vi "Main menu_3_enablepp.vi"() -> ()   [LabVIEW 2022 SP3]
uses:
  <vilib>/event_ctls.llb/lveventtype.ctl
  <vilib>/Utility/file.llb/Write Delimited Spreadsheet (DBL).vi
panel:
  in  "signal show":string(combo)
  out "Close":bool
  in  "Close app":bool
  out "Waveform Graph 2":waveform(sgl)(graph)
  in  "?":T1(tab)
  in  "New plot":bool
  in  "Multicolumn Listbox":i32(listbox)
  in  "Close All plots":bool
  in  "CSV":bool
  in  "Start":bool
  in  "Refresh time (ms)":i32
  in  "Mode":enum32{"Item 0", "Item 1"}(radio)
  in  "Size bytes":i32
  in  "Trace names":string(combo)
  out "Total\ncontrols":i32
  in  "# Control":string(combo)
  out "Current CS status":i32
  out "Enable?":bool
  in  "CS enable":bool
  in  "CS_IF_Cluster 2":T2 {"CS_Duty" min=0 max=1 scale=0.0..1.0}
  out "IP Free?":bool
  out "Server Ping":string
  out "Saved":bool
  in  "Save conf":bool
  in  "Ping IP":bool
  in  "Port":i32
  in  "hostname":string
  in  "timeout ms":i32
  in  "Send message":bool
  in  "Process 2":i32
  in  "msj":string
  # "hostname: 127.0.0.1\nport: 8085"
  # "hostname\n131.246.75.169"
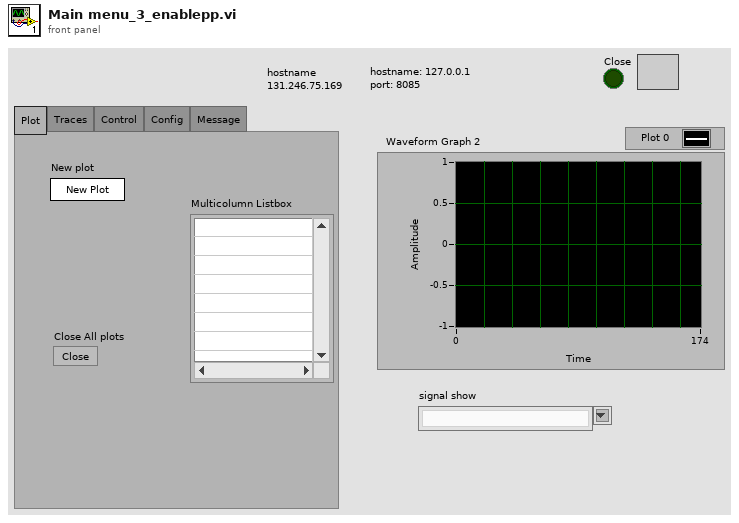
[diagram p1: front panel]
types:
  T1 = enum32{"Plot", "Traces", "Control", "Config", "Message"}
  T2 = cluster{"SET_DAMMS":i32, "CTLR":i32, "CS_Duty":sgl, "CS_IF_SET":i32}
  T3 = cluster{"Port":i32, "hostname":string, "status":bool, "timeout ms":i32, "TRACES_NAMES":string[], "Refresh time ms":i32, "Mode":enum32{"Item 0", "Item 1"}, "Start":bool, "DATA":sgl[][], "SIGNALS_NAMES":string[], "NB_SIGNALS":i32, "NB_TRACES":i32, "ID_TRACE":i32, "Mark":bool, "Counter":i32, "NAMES CSs":string[], "NB_CSs":i32}
  T4 = enum8{"Enabled", "Disabled", "Disabled and Grayed Out"}
  T5 = cluster{"TRACE_SIZE":i32, "CS_ID":i32, "TRACE ID":i32, "CMD":i32, "DATA(M)":i32}
  T6 = cluster{"timeout ms":i32, "remote port":u16, "Address":string}
  T7 = typedef "lveventtype.ctl" = enum32{"Null", "Timeout", "Annotation Menu Selection", "Annotation Menu Selection?", "App Instance Close", "App Instance Close?", "Autoscale Range Change", "Bookmark Info Change", "Cell Edit", "Cell Edit?", "Cursor Grab", "Cursor Grab?", "Cursor Menu Selection", "Cursor Menu Selection?", "Cursor Move", "Cursor Release", "Data Change", "Direction Change", "Display State Change", "Drag Ended", "Drag Enter", "Drag Leave", "Drag Over", "Drag Source Update", "Drag Starting", "Drag Starting?", "Drop", "Exec State Change", "Key Down", "Key Down?", "Key Repeat", "Key Repeat?", "Key Up", "Listbox Double Click", "Menu Activation?", "Menu Selection (App)", "Menu Selection? (App)", "Menu Selection (User)", "Mouse Down", "Mouse Down?", "Mouse Enter", "Mouse Leave", "Mouse Move", "Mouse Up", "Mouse Wheel", "NI Security User Change (App)", "Pane Size", "Panel Close", "Panel Close?", "Panel Resize", "Plot Attribute Change", "Scale Range Change", "Shortcut Menu Activation?", "Shortcut Menu Selection (App)", "Shortcut Menu Selection? (App)", "Shortcut Menu Selection (User)", "Tree Double Click", "Tree Drag", "Tree Drag?", "Tree Drop", "Tree Drop?", "Tree Item Close", "Tree Item Close?", "Tree Item Open", "Tree Item Open?", "User Event", "Value Change"}
  T8 = enum16{"open", "replace", "create", "open or create", "replace or create", "replace or create with confirmation"}
  T9 = cluster{"SIZE":i32, " TRACE DATA":sgl[], "TRACE_SIZE":i32, "NB_TRACES":i32, "NB_TRACED_SIGNALS":i32, "NAMES TRACED SIGNALS":string[], "NAMES TRACES":string[], "CS STATUS":i32, "NB_CSs":i32, "NAMES CSs":string[], "DATA (M)":sgl[], "CMD":i32}
  T10 = cluster{"SIZE":i32, "DATA":sgl[], "TRACE_SIZE":i32, "NB_TRACES":i32, "NB_SIGNALS":i32, "string":string[]}
  T11 = enum32{"invalid app kind", "Development System", "Run Time System", "Student Edition", "Embedded LabVIEW", "Evaluation", "Custom"}
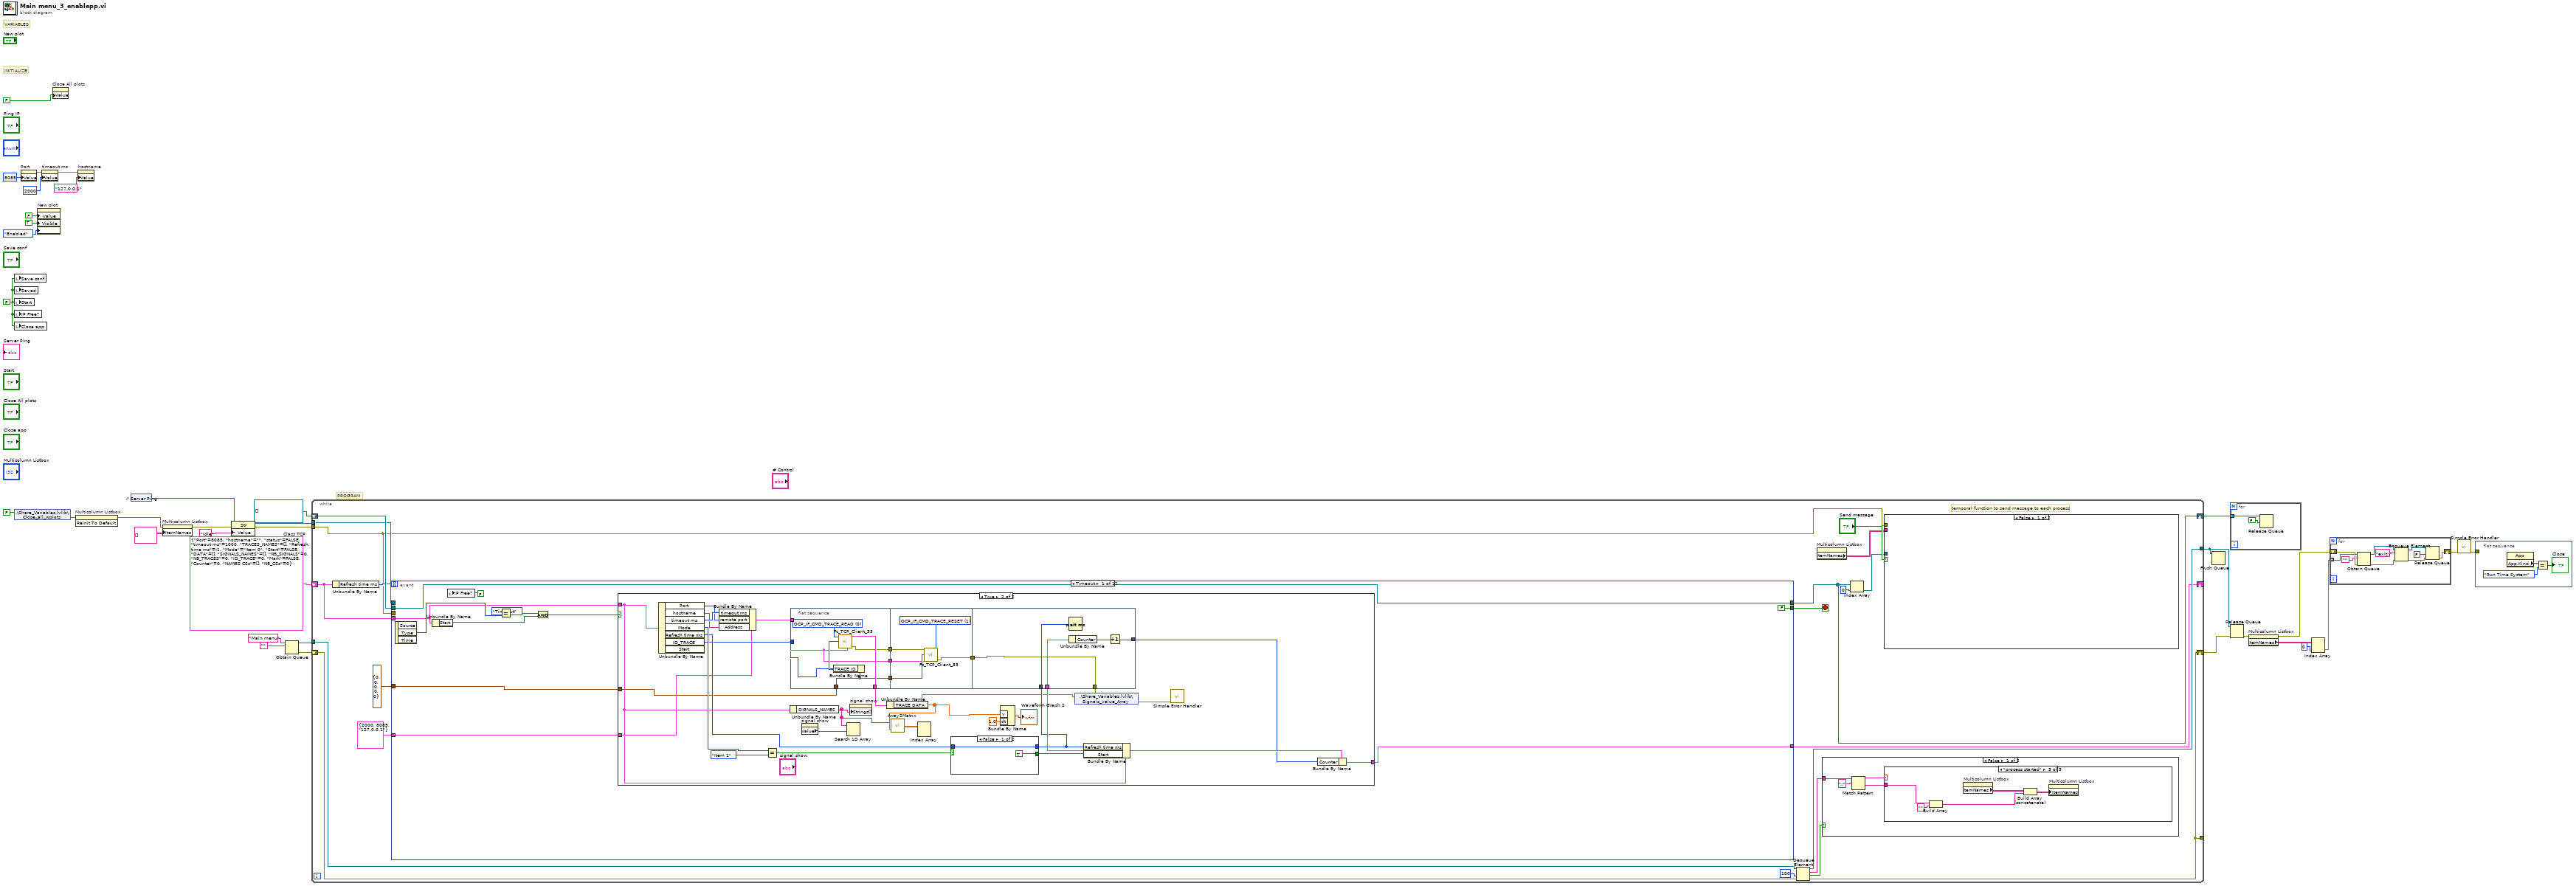
[diagram p0: block diagram]
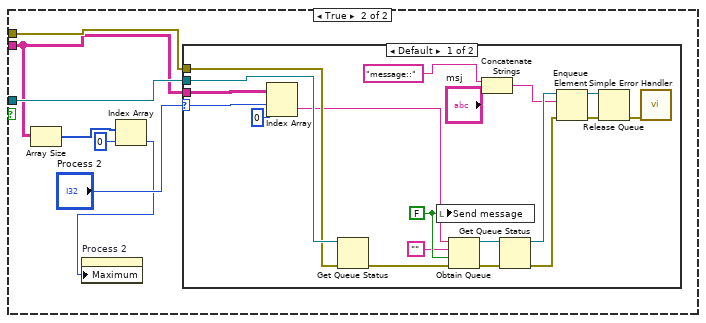
[diagram p2: hidden frame]
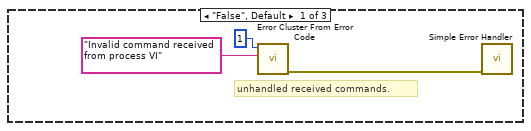
[diagram p4: hidden frame]
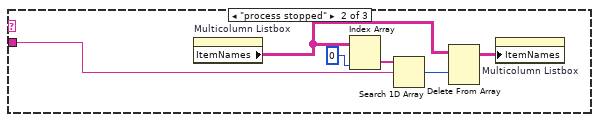
[diagram p5: hidden frame]
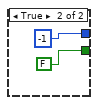
[diagram p8: hidden frame]
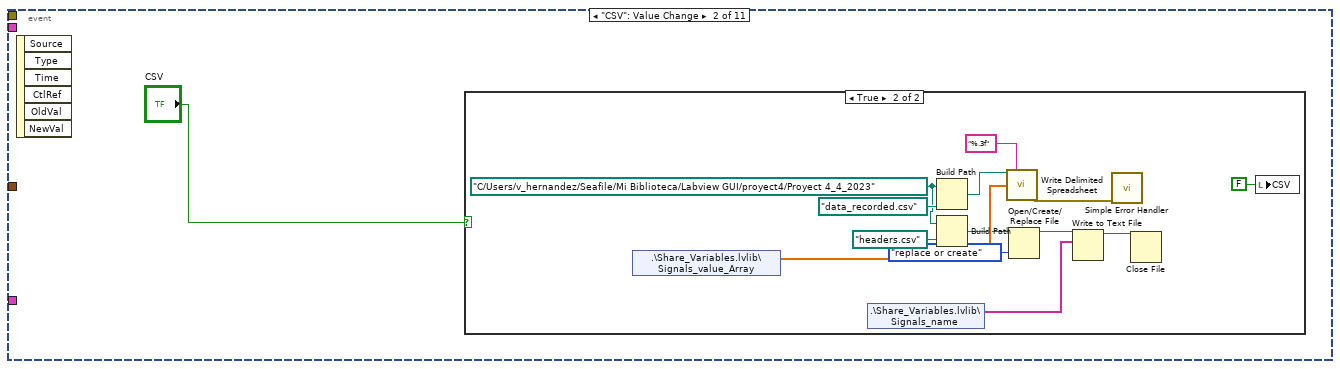
[diagram p9: hidden frame]
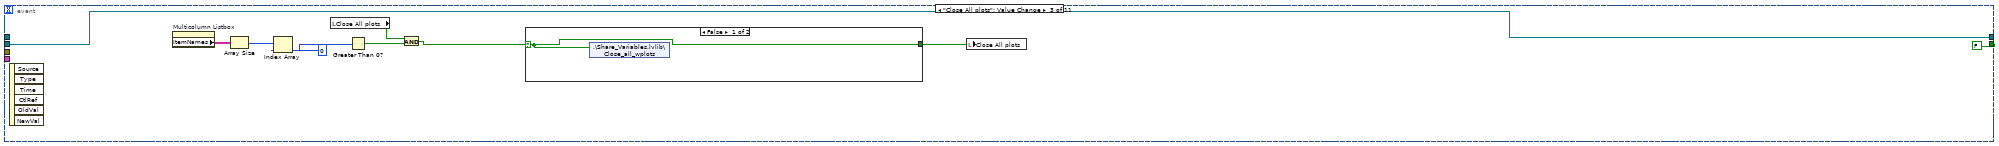
[diagram p11: hidden frame]
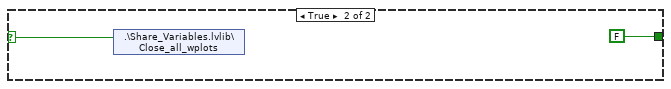
[diagram p12: hidden frame]
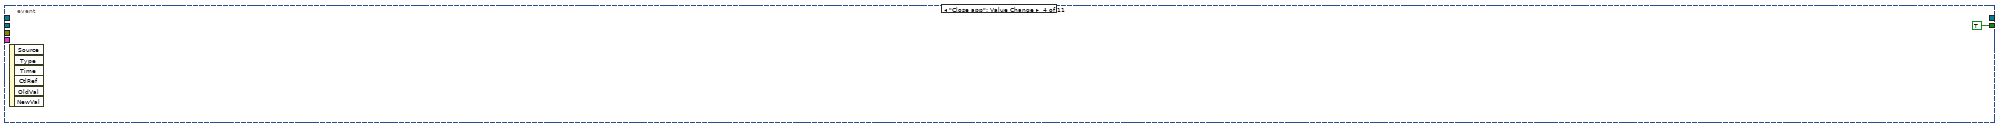
[diagram p13: hidden frame]
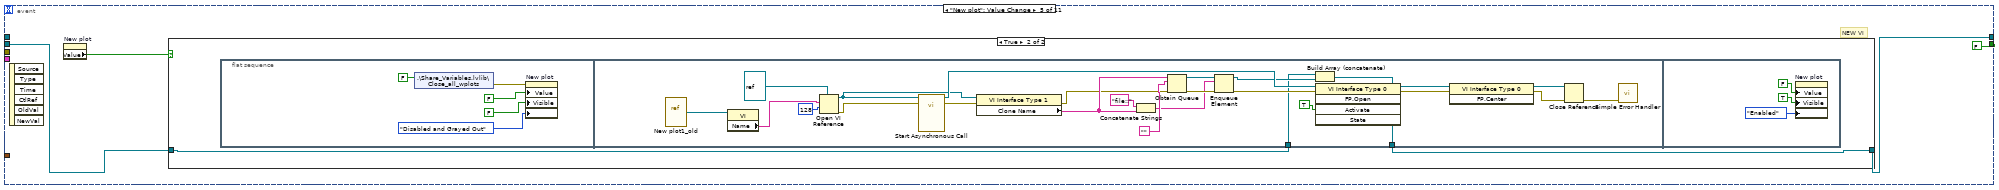
[diagram p14: hidden frame]
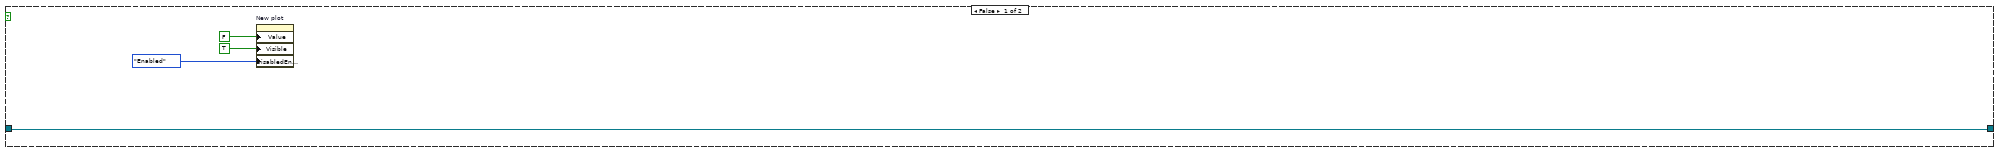
[diagram p15: hidden frame]
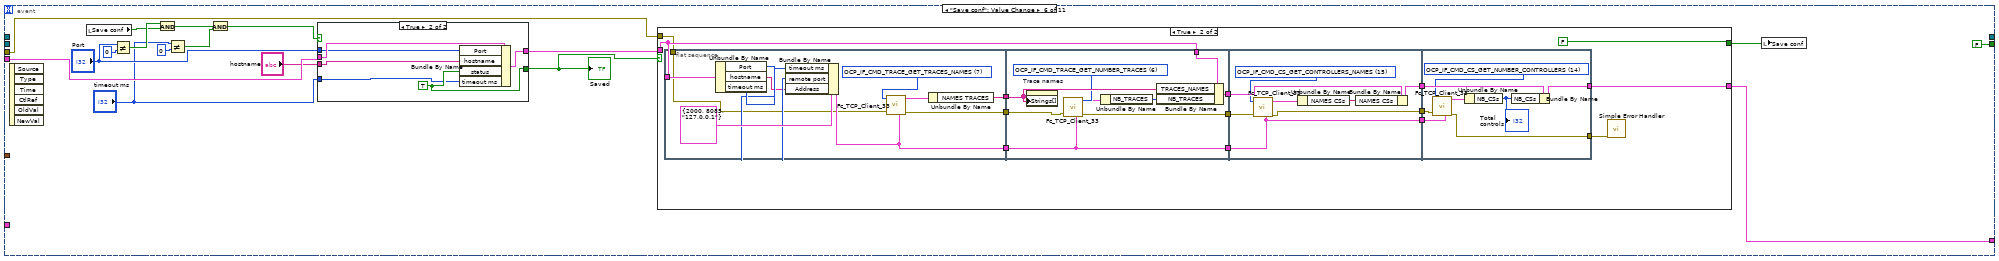
[diagram p16: hidden frame]
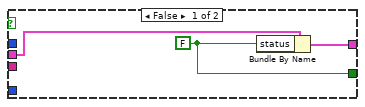
[diagram p18: hidden frame]
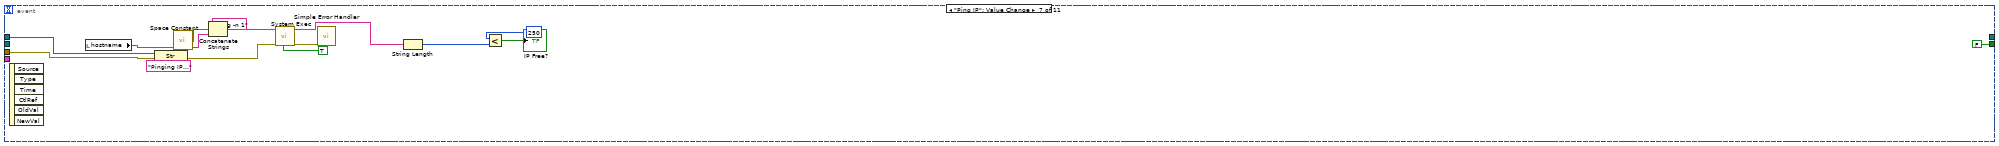
[diagram p19: hidden frame]
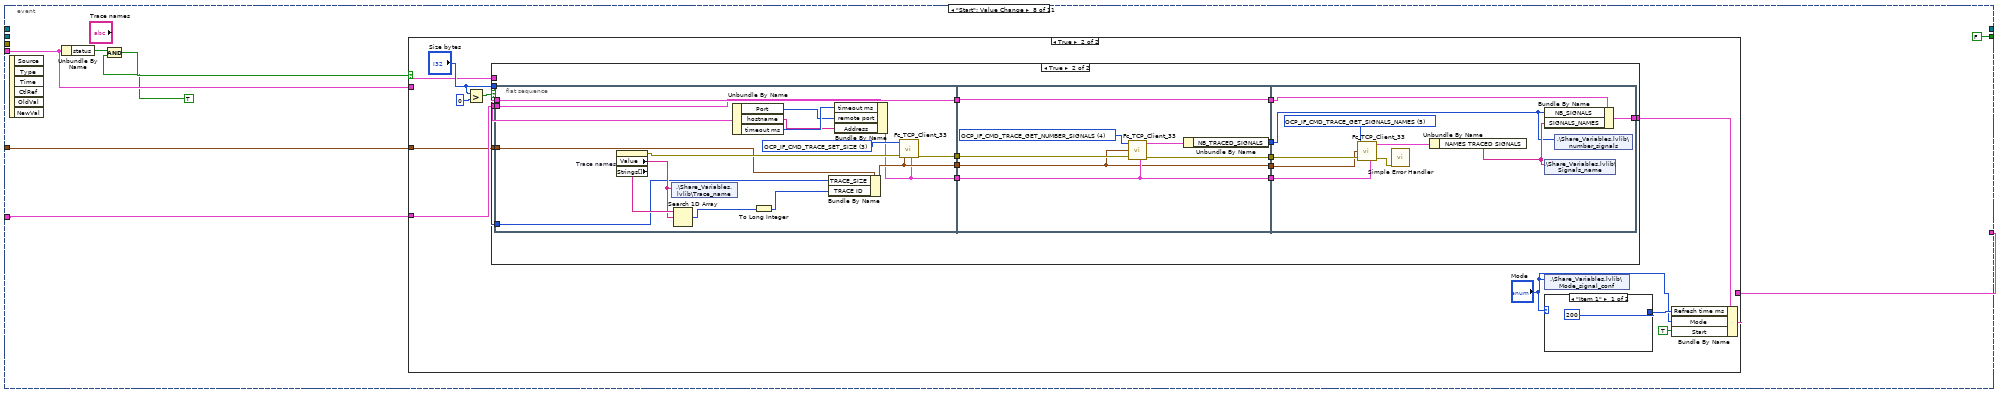
[diagram p20: hidden frame]
diagram:
  w13 = T3 {"Port"=8085, "hostname"="", "status"=FALSE, "timeout ms"=1000, "TRACES_NAMES"=[], "Refresh time ms"=-1, "Mode"=enum."Item 0", "Start"=FALSE, "DATA"=[], "SIGNALS_NAMES"=[], "NB_SIGNALS"=0, "NB_TRACES"=0, "ID_TRACE"=0, "Mark"=FALSE, "Counter"=0, "NAMES CSs"=[], "NB_CSs"=0}  # Class TCP
  w1 = FALSE ("Save conf")
  # "PROGRAM"
  # "INITIALIZE"
  # "VARIABLES"
  n1 = local write "Save conf"(w1) -> ()
  n2 = local write "Saved"(w1) -> ()
  n3 = local write "Start"(w1) -> ()
  n4 = local write "IP Free?"(w1) -> ()
  n5 = local write "Close app"(w1) -> ()
  n6 = shared-variable ".\\Share_Variables.lvlib\\Close_all_wplots"(FALSE ("Close_all_wplots")) -> (error out=w7:errorcluster)  [unwired: 1 in]
  n7 = property on="Port" class="DigNum (strict)"("Value"=8085) -> (error out=w8:errorcluster)  [unwired: 2 in, 1 out]
  n8 = property on="New plot" class="Bool (strict)"("Value"=FALSE ("New plot"), "Visible"=TRUE, "DisabledEnum"=T4."Enabled" ("Disabled")) -> ()  [unwired: 2 in, 2 out]
  n9 = property on="timeout ms" class="DigNum (strict)"(error in=w8, "Value"=2000 ("timeout ms")) -> (error out=w4:errorcluster)  [unwired: 1 in, 1 out]
  n10 = property on="Close All plots" class="Bool (strict)"("Value"=FALSE ("Cancel Button")) -> ()  [unwired: 2 in, 2 out]
  n11 = invoke on="Multicolumn Listbox" class="MCListbox (strict)" method="Reinit To Default"(error in=w7) -> (error out=w16:errorcluster)  [unwired: 2 in, 2 out]
  n12 = property on="hostname" class="Str"(error in=w4, "Value"="127.0.0.1" ("hostname")) -> ()  [unwired: 1 in, 2 out]
  n13 = control-ref of="Server Ping"() -> (w10:refnum<vi>)
  n14 = property on="Multicolumn Listbox" class="MCListbox (strict)"(error in=w16, "ItemNames"=string[][] [] ("Item Names")) -> (error out=w2:errorcluster)  [unwired: 1 in, 1 out]
  n15 = property class="Str"(reference=w10, error in=w2, "Value"="Idle" ("Ping status")) -> (reference out=w12:refnum<vi>, error out=w11:errorcluster)
  n16 = Obtain Queue(name (unnamed)="Main menu", element data type="") -> (queue out=w28:refnum<queue>, error out=w26:errorcluster)  [unwired: 3 in, 1 out]
  n17 = while {
    shift-right: [w39] -> w32
    shift-left: refnum<queue>[] [] -> [w55]
    tunnel: w28 -> [w54]
    tunnel: [w51] -> w18
    shift-right: [w44] -> w27
    shift-left: w26 -> [w50]
    shift-right: [w48] -> _
    shift-left: w13 -> [w46]
    tunnel: w12 -> [w47]
    tunnel: w11 -> [w41]
    tunnel: [w44] -> _
    stop <- w56 stop-if-true
    # "temporal function to send message to each process"
    n18 = Unbundle By Name(w46) -> ("Refresh time ms"=w45:i32)
    n19 = event shown="[0] Timeout" {
      selector: _ -> [_ _ _ _ _ _ _ _ _ _ _]
      dyn-events: _ -> [_ _ _ _ _ _ _ _ _ _ _]
      timeout: w45 -> [_ _ _ _ _ _ _ _ _ _ _]
      tunnel: [FALSE ("f") _ FALSE ("f") TRUE ("f") FALSE ("f") FALSE ("f") FALSE ("f") FALSE ("f") FALSE ("f") _ _] -> w56
      tunnel: [w112 _ w188 _ w195 _ _ _ _ _ _] -> w39
      tunnel: w55 -> [w112 _ w188 _ w194 _ _ _ _ _ _]
      tunnel: [w104 _ _ _ _ w242 _ w333 _ _ _] -> w48
      tunnel: w46 -> [w105 _ _ _ _ w250 _ w334 w414 w422 w446]
      tunnel: w47 -> [_ _ _ _ _ _ w328 _ _ _ _]
      tunnel: w41 -> [_ _ _ _ _ w245 w315 _ _ _ _]
      tunnel: T6 {"timeout ms"=2000, "remote port"=8085, "Address"="127.0.0.1"} ("Comunication Cluster") -> [w101 _ _ _ _ _ _ w330 _ w421 w445]
      tunnel: T5 {"TRACE_SIZE"=0, "CS_ID"=0, "TRACE ID"=0, "CMD"=0, "DATA(M)"=0} ("Input Cluster") -> [w102 _ _ _ _ _ _ w329 _ w420 w444]
      event Timeout {
        n20 = event-data() -> ("Type"=w109:T7)  [unwired: 1 in, 2 out]
        n21 = Unbundle By Name(w105) -> ("Start"=w107:bool)
        n22 = local write "IP Free?"(FALSE ("IP Free?")) -> ()
        n23 = Equal?(x=lveventtype."Timeout" ("Type"), y=w109) -> (x = y?=w108:bool)
        n24 = And(x=w108, y=w107) -> (x .and. y?=w106:bool)
        n25 = case shown="True" w106 {
          tunnel: w105 -> [w113 w118]
          tunnel: [w113 w133] -> w104
          tunnel: w102 -> [_ w120]
          tunnel: w101 -> [_ w119]
          frame False {
          }
          frame True {
            n26 = Unbundle By Name(w118) -> ("Port"=w125:i32, "hostname"=w124:string, "timeout ms"=w126:i32, "Mode"=w143:enum32{"Item 0", "Item 1"}, "Refresh time ms"=w140:i32, "ID_TRACE"=w137:i32)  [unwired: 1 out]
            n27 = Bundle By Name(cluster=w119, "timeout ms"=w126, "remote port"=w125, "Address"=w124) -> (w123:T6)
            n28 = Equal?(x=w143, y=enum32{"Item 0", "Item 1"}."Item 1" ("Mode")) -> (x = y?=w141:bool)
            n29 = Unbundle By Name(w118) -> ("SIGNALS_NAMES"=w116:string[])
            n30 = flat-sequence {
              tunnel: w137 -> [w146]
              tunnel: [w150] -> w136
              tunnel: [w149] -> w135
              tunnel: w120 -> [w145]
              tunnel: [w145] -> w128
              tunnel: [w144] -> w127
              tunnel: w123 -> [w144]
              tunnel: w135 -> [w155]
              tunnel: w128 -> [w154]
              tunnel: w127 -> [w153]
              tunnel: [w151] -> w122
              tunnel: w134 -> [w160]
              tunnel: [w158] -> w132
              tunnel: w130 -> [w157]
              tunnel: w122 -> [w156]
              tunnel: [w156] -> w121
              frame #0 {
                w148 = 0 items=["OCP_IF_CMD_TRACE_READ", "OCP_IF_CMD_TRACE_RESET", "OCP_IF_CMD_TRACE_GET_SIZE", "OCP_IF_CMD_TRACE_SET_SIZE", "OCP_IF_CMD_TRACE_GET_NUMBER_SIGNALS", "OCP_IF_CMD_TRACE_GET_SIGNALS_NAMES", "OCP_IF_CMD_TRACE_GET_NUMBER_TRACES", "OCP_IF_CMD_TRACE_GET_TRACES_NAMES", "OCP_IF_CMD_TRACE_GET_ADDRESS", "OCP_IF_CMD_CS_STATUS", "OCP_IF_CMD_CS_ENABLE", "OCP_IF_CMD_CS_DISABLE", "OCP_IF_CMD_CS_CONTROLLER_IF", "OCP_IF_CMD_CS_HARDWARE_IF", "OCP_IF_CMD_CS_GET_NUMBER_CONTROLLERS", "OCP_IF_CMD_CS_GET_CONTROLLERS_NAMES", "OCP_IF_CMD_PLATFORM_ID", "OCP_IF_CMD_PLATFORM_IF", "OCP_IF_CMD_OPIL_UPDATE_MEASUREMENTS", "OCP_IF_CMD_OPIL_UPDATE_SIM_DATA", "OCP_IF_CMD_OPIL_RUN_CONTROL", "OCP_IF_CMD_OPIL_INITIALIZE_CONTROL", "OCP_IF_CMD_OPIL_GET_CONTROL", "OCP_IF_CMD_OPIL_GET_CONTROLLER_DATA", "OCP_IF_CMD_END"] ("CMD")
                n31 = Bundle By Name(cluster=w145, "TRACE ID"=w146) -> (w147:T5)
                n32 = call "Fc_TCP_Client_33.vi"("CMD"=w148, "Input Cluster"=w147, "Comunication Cluster"=w144) -> ("Output cluster"=w150:T9, "error out"=w149:errorcluster)  [unwired: 5 in, 1 out]
              }
              frame #1 {
                w152 = 1 items=["OCP_IF_CMD_TRACE_READ", "OCP_IF_CMD_TRACE_RESET", "OCP_IF_CMD_TRACE_GET_SIZE", "OCP_IF_CMD_TRACE_SET_SIZE", "OCP_IF_CMD_TRACE_GET_NUMBER_SIGNALS", "OCP_IF_CMD_TRACE_GET_SIGNALS_NAMES", "OCP_IF_CMD_TRACE_GET_NUMBER_TRACES", "OCP_IF_CMD_TRACE_GET_TRACES_NAMES", "OCP_IF_CMD_TRACE_GET_ADDRESS", "OCP_IF_CMD_CS_STATUS", "OCP_IF_CMD_CS_ENABLE", "OCP_IF_CMD_CS_DISABLE", "OCP_IF_CMD_CS_CONTROLLER_IF", "OCP_IF_CMD_CS_HARDWARE_IF", "OCP_IF_CMD_CS_GET_NUMBER_CONTROLLERS", "OCP_IF_CMD_CS_GET_CONTROLLERS_NAMES", "OCP_IF_CMD_PLATFORM_ID", "OCP_IF_CMD_PLATFORM_IF", "OCP_IF_CMD_OPIL_UPDATE_MEASUREMENTS", "OCP_IF_CMD_OPIL_UPDATE_SIM_DATA", "OCP_IF_CMD_OPIL_RUN_CONTROL", "OCP_IF_CMD_OPIL_INITIALIZE_CONTROL", "OCP_IF_CMD_OPIL_GET_CONTROL", "OCP_IF_CMD_OPIL_GET_CONTROLLER_DATA", "OCP_IF_CMD_END"] ("CMD")
                n33 = call "Fc_TCP_Client_33.vi"("CMD"=w152, "Input Cluster"=w154, "error in (no error)"=w155, "Comunication Cluster"=w153) -> ("error out"=w151:errorcluster)  [unwired: 4 in, 2 out]
              }
              frame #2 {
                n34 = Wait (ms)(milliseconds to wait=w157) -> ()  [unwired: 1 out]
                n35 = Unbundle By Name(w160) -> ("Counter"=w159:i32)
                n36 = Increment(x=w159) -> (x+1=w158:i32)
              }
            }
            n37 = property on="signal show" class="CmbBox"() -> ("Value"=w115:string)  [unwired: 2 in, 2 out]
            n38 = Search 1D Array(1D array=w116, element=w115) -> ()  [unwired: 1 in, 1 out]
            n39 = property on="signal show" class="CmbBox"("Strings[]"=w116) -> ()  [unwired: 2 in, 2 out]
            n40 = Unbundle By Name(w136) -> ("TRACE DATA"=w117:sgl[])
            n41 = call "Array2Matrix.vi"("Array"=w117, "Header"=w116) -> ("Array2D"=w114:sgl[][])
            n42 = Index Array(array=w114) -> ()  [unwired: 2 in, 1 out]
            n43 = case shown="False" w141 {
              tunnel: [TRUE FALSE] -> w139
              tunnel: [w161 i8 -1 ("t")] -> w130
              tunnel: w140 -> [w161 _]
              frame False {
              }
              frame True {
              }
            }
            n44 = Bundle By Name("Y"=w117, "dt"=1.0) -> (→"Waveform Graph 2":waveform(sgl))  [unwired: 1 in]
            n45 = shared-variable ".\\Share_Variables.lvlib\\Signals_value_Array"(w117, error in=w121) -> (error out=w138:errorcluster)
            n46 = Bundle By Name(cluster=w118, "Refresh time ms"=w130, "Start"=w139) -> (w134:T3)
            n47 = call <vilib>:"Simple Error Handler.vi"("error in (no error)"=w138) -> ()  [unwired: 4 in, 5 out]
            n48 = Bundle By Name(cluster=w134, "Counter"=w132) -> (w133:T3)
          }
        }
      }
      event "CSV": Value Change {
        n49 = event-data() -> ()  [unwired: 1 in, 6 out]
        n50 = case shown="True" "CSV" {
          frame False {
          }
          frame True {
            w173 = path "C:/Users/v_hernandez/Seafile/Mi Biblioteca/Labview GUI/proyect4/Proyect 4_4_2023" ("base path")
            n51 = shared-variable ".\\Share_Variables.lvlib\\Signals_value_Array"() -> (w175:dbl[])  [unwired: 1 in, 1 out]
            n52 = shared-variable ".\\Share_Variables.lvlib\\Signals_name"() -> (w168:string[])  [unwired: 1 in, 1 out]
            n53 = Build Path(base path=w173, name or relative path=path "data_recorded.csv") -> (appended path=w174:path)
            n54 = Build Path(base path=w173, name or relative path=path "headers.csv") -> (appended path=w171:path)
            n55 = call-poly <vilib>:"Write Delimited Spreadsheet.vi"("file path (dialog if empty)"=w174, "format (%.3f)"="%.3f", "1D data"=w175) -> ("error out"=w176:errorcluster)  [unwired: 11 in, 1 out]
            n56 = Open/Create/Replace File(file path (use dialog)=w171, operation (0:open)=T8."replace or create") -> (refnum out=w169:refnum<file>)  [unwired: 4 in, 2 out]
            n57 = Write to Text File(file (use dialog)=w169, text=w168) -> (refnum out=w167:refnum<file>)  [unwired: 2 in, 2 out]
            n58 = call <vilib>:"Simple Error Handler.vi"("error in (no error)"=w176) -> ()  [unwired: 4 in, 5 out]
            n59 = Close File(refnum=w167) -> ()  [unwired: 1 in, 2 out]
            n60 = local write "CSV"(FALSE ("CSV")) -> ()
          }
        }
      }
      event "Close All plots": Value Change {
        n61 = event-data() -> ()  [unwired: 1 in, 6 out]
        n62 = property on="Multicolumn Listbox" class="MCListbox (strict)"() -> ("ItemNames"=w182:string[][])  [unwired: 2 in, 2 out]
        n63 = Array Size(array=w182) -> (size(s)=w186:i32[])
        n64 = Index Array(array=w186, index=0) -> (element=w184:i32)
        n65 = local read "Close All plots"() -> (w181:bool)
        n66 = Greater Than 0?(x=w184) -> (x > 0?=w179:bool)
        n67 = And(x=w181, y=w179) -> (x .and. y?=w180:bool)
        n68 = case shown="False" w180 {
          selector: w180 -> [w189 w190]
          tunnel: [w189 FALSE] -> w183
          frame False {
            n69 = shared-variable ".\\Share_Variables.lvlib\\Close_all_wplots"(w189) -> ()  [unwired: 1 in, 1 out]
          }
          frame True {
            n70 = shared-variable ".\\Share_Variables.lvlib\\Close_all_wplots"(w190) -> ()  [unwired: 1 in, 1 out]
          }
        }
        n71 = local write "Close All plots"(w183) -> ()
      }
      event "Close app": Value Change {
        n72 = event-data() -> ()  [unwired: 1 in, 6 out]
      }
      event "New plot": Value Change {
        # "NEW VI"
        n73 = event-data() -> ()  [unwired: 1 in, 6 out]
        n74 = property on="New plot" class="Bool (strict)"() -> ("Value"=w196:bool)  [unwired: 2 in, 2 out]
        n75 = case shown="True" w196 {
          tunnel: [w197 w202] -> w195
          tunnel: w194 -> [w197 w201]
          frame False {
            n76 = property on="New plot" class="Bool (strict)"("Value"=FALSE ("New plot"), "Visible"=TRUE, "DisabledEnum"=T4."Enabled" ("Disabled")) -> ()  [unwired: 2 in, 2 out]
          }
          frame True {
            n77 = flat-sequence {
              tunnel: [w213] -> w202
              tunnel: w201 -> [w212]
              frame #0 {
                n78 = shared-variable ".\\Share_Variables.lvlib\\Close_all_wplots"(FALSE ("Close_all_wplots")) -> (error out=w203:errorcluster)  [unwired: 1 in]
                n79 = property on="New plot" class="Bool (strict)"(error in=w203, "Value"=FALSE ("New plot"), "Visible"=FALSE, "DisabledEnum"=T4."Disabled and Grayed Out" ("Disabled")) -> ()  [unwired: 1 in, 2 out]
              }
              frame #1 {
                n80 = vi-ref "New plot1_old.vi"() -> (w226:refnum<vi>)
                n81 = property class="VI"(reference=w226) -> ("Name"=w232:string)  [unwired: 1 in, 2 out]
                n82 = Open VI Reference(type specifier VI Refnum (for type only)=refnum<vi> refnum, vi path=w232, options=128) -> (vi reference=w223:refnum<vi>, error out=w228:errorcluster)  [unwired: 3 in]
                n83 = call-by-ref "Start Asynchronous Call"(reference=w223, error in=w228) -> (reference out=w227:refnum<vi>, error out=w217:errorcluster)  [unwired: 1 in, 1 out]
                n84 = property class="VI Interface Type 1"(reference=w223, error in=w217) -> (error out=w218:errorcluster, "Clone Name"=w220:string)  [unwired: 1 out]
                n85 = Concatenate Strings("file::" ("string"), w220) -> (w211:string)
                n86 = Obtain Queue(name (unnamed)=w220, element data type="", error in (no error)=w218) -> (queue out=w219:refnum<queue>, error out=w216:errorcluster)  [unwired: 2 in, 1 out]
                n87 = Enqueue Element(queue=w219, element=w211, error in (no error)=w216) -> (queue out=w214:refnum<queue>, error out=w215:errorcluster)  [unwired: 1 in, 1 out]
                n88 = Build Array (concatenate)(w212, w214) -> (w213:refnum<queue>[])
                n89 = invoke class="VI Interface Type 0" method="FP.Open"(reference=w227, error in=w215, "Activate"=TRUE ("Activate?")) -> (reference out=w225:refnum<vi>, error out=w210:errorcluster)  [unwired: 2 in, 3 out]
                n90 = invoke class="VI Interface Type 0" method="FP.Center"(reference=w225, error in=w210) -> (reference out=w224:refnum<vi>, error out=w209:errorcluster)  [unwired: 1 in, 1 out]
                n91 = Close Reference(reference=w224, error in (no error)=w209) -> (error out=w208:errorcluster)
                n92 = call <vilib>:"Simple Error Handler.vi"("error in (no error)"=w208) -> ()  [unwired: 4 in, 5 out]
              }
              frame #2 {
                n93 = property on="New plot" class="Bool (strict)"("Value"=FALSE ("Value (Signaling)"), "Visible"=TRUE, "DisabledEnum"=T4."Enabled" ("Disabled")) -> ()  [unwired: 2 in, 2 out]
              }
            }
          }
        }
      }
      event "Save conf": Value Change {
        n94 = event-data() -> ()  [unwired: 1 in, 6 out]
        n95 = local read "Save conf"() -> (w247:bool)
        n96 = Not Equal?(x="Port", y=0) -> (x != y?=w251:bool)
        n97 = And(x=w251, y=w247) -> (x .and. y?=w237:bool)
        n98 = Not Equal?(x="timeout ms", y=0) -> (x != y?=w239:bool)
        n99 = And(x=w237, y=w239) -> (x .and. y?=w238:bool)
        n100 = case shown="True" w238 {
          tunnel: [w305 w310] -> w246
          tunnel: "Port" -> [_ w312]
          tunnel: "hostname" -> [_ w311]
          tunnel: [w307 w308] -> w243
          tunnel: w250 -> [w306 w313]
          tunnel: "timeout ms" -> [_ w309]
          frame False {
            w305 = FALSE
            n101 = Bundle By Name(cluster=w306, "status"=w305) -> (w307:T3)
          }
          frame True {
            w310 = TRUE
            n102 = Bundle By Name(cluster=w313, "Port"=w312, "hostname"=w311, "status"=w310, "timeout ms"=w309) -> (w308:T3)
          }
        }
        "Saved" <- w246
        n103 = case shown="True" w246 {
          selector: w246 -> [w253 _]
          tunnel: w245 -> [_ w256]
          tunnel: [w253 FALSE] -> w244
          tunnel: w243 -> [w254 w267]
          tunnel: [w254 w266] -> w242
          frame False {
          }
          frame True {
            n104 = flat-sequence {
              tunnel: w267 -> [w279]
              tunnel: [w272] -> w265
              tunnel: [w271] -> w264
              tunnel: [w270] -> w263
              tunnel: w256 -> [w269]
              tunnel: w267 -> [w288]
              tunnel: w265 -> [w285]
              tunnel: w264 -> [w284]
              tunnel: w263 -> [w280]
              tunnel: [w287] -> w262
              tunnel: [w281] -> w260
              tunnel: [w280] -> w259
              tunnel: w262 -> [w296]
              tunnel: [w290] -> w261
              tunnel: w260 -> [w295]
              tunnel: w259 -> [w292]
              tunnel: [w293] -> w258
              tunnel: [w292] -> w257
              tunnel: [w300] -> w266
              tunnel: w261 -> [w304]
              tunnel: w258 -> [w303]
              tunnel: w257 -> [w302]
              tunnel: [w298] -> w255
              frame #0 {
                w278 = 7 items=["OCP_IF_CMD_TRACE_READ", "OCP_IF_CMD_TRACE_RESET", "OCP_IF_CMD_TRACE_GET_SIZE", "OCP_IF_CMD_TRACE_SET_SIZE", "OCP_IF_CMD_TRACE_GET_NUMBER_SIGNALS", "OCP_IF_CMD_TRACE_GET_SIGNALS_NAMES", "OCP_IF_CMD_TRACE_GET_NUMBER_TRACES", "OCP_IF_CMD_TRACE_GET_TRACES_NAMES", "OCP_IF_CMD_TRACE_GET_ADDRESS", "OCP_IF_CMD_CS_STATUS", "OCP_IF_CMD_CS_ENABLE", "OCP_IF_CMD_CS_DISABLE", "OCP_IF_CMD_CS_CONTROLLER_IF", "OCP_IF_CMD_CS_HARDWARE_IF", "OCP_IF_CMD_CS_GET_NUMBER_CONTROLLERS", "OCP_IF_CMD_CS_GET_CONTROLLERS_NAMES", "OCP_IF_CMD_PLATFORM_ID", "OCP_IF_CMD_PLATFORM_IF", "OCP_IF_CMD_OPIL_UPDATE_MEASUREMENTS", "OCP_IF_CMD_OPIL_UPDATE_SIM_DATA", "OCP_IF_CMD_OPIL_RUN_CONTROL", "OCP_IF_CMD_OPIL_INITIALIZE_CONTROL", "OCP_IF_CMD_OPIL_GET_CONTROL", "OCP_IF_CMD_OPIL_GET_CONTROLLER_DATA", "OCP_IF_CMD_END"] ("CMD")
                n105 = Unbundle By Name(w279) -> ("Port"=w274:i32, "hostname"=w273:string, "timeout ms"=w275:i32)
                n106 = Bundle By Name(cluster=T6 {"timeout ms"=2000, "remote port"=8085, "Address"="127.0.0.1"} ("Comunication Cluster"), "timeout ms"=w275, "remote port"=w274, "Address"=w273) -> (w270:T6)
                n107 = call "Fc_TCP_Client_33.vi"("CMD"=w278, "error in (no error)"=w269, "Comunication Cluster"=w270) -> ("Output cluster"=w277:T9, "error out"=w271:errorcluster)  [unwired: 5 in, 1 out]
                n108 = Unbundle By Name(w277) -> ("NAMES TRACES"=w272:string[])
              }
              frame #1 {
                w283 = 6 items=["OCP_IF_CMD_TRACE_READ", "OCP_IF_CMD_TRACE_RESET", "OCP_IF_CMD_TRACE_GET_SIZE", "OCP_IF_CMD_TRACE_SET_SIZE", "OCP_IF_CMD_TRACE_GET_NUMBER_SIGNALS", "OCP_IF_CMD_TRACE_GET_SIGNALS_NAMES", "OCP_IF_CMD_TRACE_GET_NUMBER_TRACES", "OCP_IF_CMD_TRACE_GET_TRACES_NAMES", "OCP_IF_CMD_TRACE_GET_ADDRESS", "OCP_IF_CMD_CS_STATUS", "OCP_IF_CMD_CS_ENABLE", "OCP_IF_CMD_CS_DISABLE", "OCP_IF_CMD_CS_CONTROLLER_IF", "OCP_IF_CMD_CS_HARDWARE_IF", "OCP_IF_CMD_CS_GET_NUMBER_CONTROLLERS", "OCP_IF_CMD_CS_GET_CONTROLLERS_NAMES", "OCP_IF_CMD_PLATFORM_ID", "OCP_IF_CMD_PLATFORM_IF", "OCP_IF_CMD_OPIL_UPDATE_MEASUREMENTS", "OCP_IF_CMD_OPIL_UPDATE_SIM_DATA", "OCP_IF_CMD_OPIL_RUN_CONTROL", "OCP_IF_CMD_OPIL_INITIALIZE_CONTROL", "OCP_IF_CMD_OPIL_GET_CONTROL", "OCP_IF_CMD_OPIL_GET_CONTROLLER_DATA", "OCP_IF_CMD_END"] ("CMD")
                n109 = property on="Trace names" class="CmbBox"("Strings[]"=w285) -> ()  [unwired: 2 in, 2 out]
                n110 = call "Fc_TCP_Client_33.vi"("CMD"=w283, "error in (no error)"=w284, "Comunication Cluster"=w280) -> ("Output cluster"=w282:T9, "error out"=w281:errorcluster)  [unwired: 5 in, 1 out]
                n111 = Unbundle By Name(w282) -> ("NB_TRACES"=w286:i32)
                n112 = Bundle By Name(cluster=w288, "TRACES_NAMES"=w285, "NB_TRACES"=w286) -> (w287:T3)
              }
              frame #2 {
                w294 = 15 items=["OCP_IF_CMD_TRACE_READ", "OCP_IF_CMD_TRACE_RESET", "OCP_IF_CMD_TRACE_GET_SIZE", "OCP_IF_CMD_TRACE_SET_SIZE", "OCP_IF_CMD_TRACE_GET_NUMBER_SIGNALS", "OCP_IF_CMD_TRACE_GET_SIGNALS_NAMES", "OCP_IF_CMD_TRACE_GET_NUMBER_TRACES", "OCP_IF_CMD_TRACE_GET_TRACES_NAMES", "OCP_IF_CMD_TRACE_GET_ADDRESS", "OCP_IF_CMD_CS_STATUS", "OCP_IF_CMD_CS_ENABLE", "OCP_IF_CMD_CS_DISABLE", "OCP_IF_CMD_CS_CONTROLLER_IF", "OCP_IF_CMD_CS_HARDWARE_IF", "OCP_IF_CMD_CS_GET_NUMBER_CONTROLLERS", "OCP_IF_CMD_CS_GET_CONTROLLERS_NAMES", "OCP_IF_CMD_PLATFORM_ID", "OCP_IF_CMD_PLATFORM_IF", "OCP_IF_CMD_OPIL_UPDATE_MEASUREMENTS", "OCP_IF_CMD_OPIL_UPDATE_SIM_DATA", "OCP_IF_CMD_OPIL_RUN_CONTROL", "OCP_IF_CMD_OPIL_INITIALIZE_CONTROL", "OCP_IF_CMD_OPIL_GET_CONTROL", "OCP_IF_CMD_OPIL_GET_CONTROLLER_DATA", "OCP_IF_CMD_END"] ("CMD")
                n113 = call "Fc_TCP_Client_33.vi"("CMD"=w294, "error in (no error)"=w295, "Comunication Cluster"=w292) -> ("Output cluster"=w291:T9, "error out"=w293:errorcluster)  [unwired: 5 in, 1 out]
                n114 = Unbundle By Name(w291) -> ("NAMES CSs"=w289:string[])
                n115 = Bundle By Name(cluster=w296, "NAMES CSs"=w289) -> (w290:T3)
              }
              frame #3 {
                w301 = 14 items=["OCP_IF_CMD_TRACE_READ", "OCP_IF_CMD_TRACE_RESET", "OCP_IF_CMD_TRACE_GET_SIZE", "OCP_IF_CMD_TRACE_SET_SIZE", "OCP_IF_CMD_TRACE_GET_NUMBER_SIGNALS", "OCP_IF_CMD_TRACE_GET_SIGNALS_NAMES", "OCP_IF_CMD_TRACE_GET_NUMBER_TRACES", "OCP_IF_CMD_TRACE_GET_TRACES_NAMES", "OCP_IF_CMD_TRACE_GET_ADDRESS", "OCP_IF_CMD_CS_STATUS", "OCP_IF_CMD_CS_ENABLE", "OCP_IF_CMD_CS_DISABLE", "OCP_IF_CMD_CS_CONTROLLER_IF", "OCP_IF_CMD_CS_HARDWARE_IF", "OCP_IF_CMD_CS_GET_NUMBER_CONTROLLERS", "OCP_IF_CMD_CS_GET_CONTROLLERS_NAMES", "OCP_IF_CMD_PLATFORM_ID", "OCP_IF_CMD_PLATFORM_IF", "OCP_IF_CMD_OPIL_UPDATE_MEASUREMENTS", "OCP_IF_CMD_OPIL_UPDATE_SIM_DATA", "OCP_IF_CMD_OPIL_RUN_CONTROL", "OCP_IF_CMD_OPIL_INITIALIZE_CONTROL", "OCP_IF_CMD_OPIL_GET_CONTROL", "OCP_IF_CMD_OPIL_GET_CONTROLLER_DATA", "OCP_IF_CMD_END"] ("CMD")
                n116 = call "Fc_TCP_Client_33.vi"("CMD"=w301, "error in (no error)"=w303, "Comunication Cluster"=w302) -> ("Output cluster"=w299:T9, "error out"=w298:errorcluster)  [unwired: 5 in, 1 out]
                n117 = Unbundle By Name(w299) -> ("NB_CSs"=w297:i32)
                "Total\ncontrols" <- w297
                n118 = Bundle By Name(cluster=w304, "NB_CSs"=w297) -> (w300:T3)
              }
            }
            n119 = call <vilib>:"Simple Error Handler.vi"("error in (no error)"=w255) -> ()  [unwired: 4 in, 5 out]
          }
        }
        n120 = local write "Save conf"(w244) -> ()
      }
      event "Ping IP": Value Change {
        n121 = event-data() -> ()  [unwired: 1 in, 6 out]
        n122 = local read "hostname"() -> (w323:string)
        n123 = property class="Str"(reference=w328, error in=w315, "Value"="Pinging IP...") -> (error out=w326:errorcluster)  [unwired: 1 out]
        n124 = call <vilib>:"Space Constant.vi"() -> ("String"=w324:string)
        n125 = Concatenate Strings("ping -n 1" ("Value"), w324, w323) -> (w322:string)
        n126 = call <vilib>:"System Exec.vi"("run minimized? (F)"=TRUE, "error in (no error)"=w326, "command line"=w322) -> ("error out"=w316:errorcluster, "standard output"=w320:string)  [unwired: 5 in, 2 out]
        n127 = call <vilib>:"Simple Error Handler.vi"("error in (no error)"=w316) -> ()  [unwired: 4 in, 5 out]
        n128 = String Length(string=w320) -> (length=w321:i32)
        n129 = Less?(x=250, y=w321) -> (x < y?=→"IP Free?":bool)
      }
      event "Start": Value Change {
        n130 = event-data() -> ()  [unwired: 1 in, 6 out]
        n131 = Unbundle By Name(w334) -> ("status"=w336:bool)
        n132 = And(x=w336, y=TRUE) -> (x .and. y?=w335:bool)
        n133 = case shown="True" w335 {
          tunnel: w334 -> [w337 w342]
          tunnel: [w337 w348] -> w333
          tunnel: w330 -> [_ w339]
          tunnel: w329 -> [_ w338]
          frame False {
          }
          frame True {
            n134 = Greater?(x="Size bytes", y=0) -> (0:w344:bool)
            n135 = case shown="True" w344 {
              tunnel: "Size bytes" -> [_ w363]
              tunnel: w342 -> [w349 w362]
              tunnel: [w349 w358] -> w341
              tunnel: w339 -> [_ w351]
              tunnel: w338 -> [_ w350]
              frame False {
              }
              frame True {
                n136 = flat-sequence {
                  tunnel: w363 -> [w369]
                  tunnel: w362 -> [w379]
                  tunnel: [w375] -> w361
                  tunnel: [w379] -> w360
                  tunnel: [w367] -> w357
                  tunnel: [w366] -> w356
                  tunnel: w351 -> [w365]
                  tunnel: w350 -> [w364]
                  tunnel: w361 -> [w386]
                  tunnel: w360 -> [w387]
                  tunnel: [w387] -> w359
                  tunnel: w357 -> [w380]
                  tunnel: w356 -> [w381]
                  tunnel: [w383] -> w355
                  tunnel: [w382] -> w354
                  tunnel: [w381] -> w353
                  tunnel: [w380] -> w352
                  tunnel: w359 -> [w397]
                  tunnel: [w396] -> w358
                  tunnel: w355 -> [w388]
                  tunnel: w354 -> [w392]
                  tunnel: w353 -> [w390]
                  tunnel: w352 -> [w389]
                  frame #0 {
                    w374 = 3 items=["OCP_IF_CMD_TRACE_READ", "OCP_IF_CMD_TRACE_RESET", "OCP_IF_CMD_TRACE_GET_SIZE", "OCP_IF_CMD_TRACE_SET_SIZE", "OCP_IF_CMD_TRACE_GET_NUMBER_SIGNALS", "OCP_IF_CMD_TRACE_GET_SIGNALS_NAMES", "OCP_IF_CMD_TRACE_GET_NUMBER_TRACES", "OCP_IF_CMD_TRACE_GET_TRACES_NAMES", "OCP_IF_CMD_TRACE_GET_ADDRESS", "OCP_IF_CMD_CS_STATUS", "OCP_IF_CMD_CS_ENABLE", "OCP_IF_CMD_CS_DISABLE", "OCP_IF_CMD_CS_CONTROLLER_IF", "OCP_IF_CMD_CS_HARDWARE_IF", "OCP_IF_CMD_CS_GET_NUMBER_CONTROLLERS", "OCP_IF_CMD_CS_GET_CONTROLLERS_NAMES", "OCP_IF_CMD_PLATFORM_ID", "OCP_IF_CMD_PLATFORM_IF", "OCP_IF_CMD_OPIL_UPDATE_MEASUREMENTS", "OCP_IF_CMD_OPIL_UPDATE_SIM_DATA", "OCP_IF_CMD_OPIL_RUN_CONTROL", "OCP_IF_CMD_OPIL_INITIALIZE_CONTROL", "OCP_IF_CMD_OPIL_GET_CONTROL", "OCP_IF_CMD_OPIL_GET_CONTROLLER_DATA", "OCP_IF_CMD_END"] ("CMD")
                    n137 = property on="Trace names" class="CmbBox"() -> (error out=w370:errorcluster, "Value"=w376:string, "Strings[]"=w378:string[])  [unwired: 2 in, 1 out]
                    n138 = shared-variable ".\\Share_Variables.lvlib\\Trace_name"(w376) -> ()  [unwired: 1 in, 1 out]
                    n139 = Search 1D Array(1D array=w378, element=w376) -> (index of element=w377:i32)  [unwired: 1 in]
                    n140 = Unbundle By Name(w379) -> ("Port"=w372:i32, "hostname"=w371:string, "timeout ms"=w373:i32)
                    n141 = To Long Integer(number=w377) -> (32bit integer=w368:i32)
                    n142 = Bundle By Name(cluster=w364, "TRACE_SIZE"=w369, "TRACE ID"=w368) -> (w367:T5)
                    n143 = Bundle By Name(cluster=w365, "timeout ms"=w373, "remote port"=w372, "Address"=w371) -> (w366:T6)
                    n144 = call "Fc_TCP_Client_33.vi"("CMD"=w374, "Input Cluster"=w367, "error in (no error)"=w370, "Comunication Cluster"=w366) -> ("error out"=w375:errorcluster)  [unwired: 4 in, 2 out]
                  }
                  frame #1 {
                    w385 = 4 items=["OCP_IF_CMD_TRACE_READ", "OCP_IF_CMD_TRACE_RESET", "OCP_IF_CMD_TRACE_GET_SIZE", "OCP_IF_CMD_TRACE_SET_SIZE", "OCP_IF_CMD_TRACE_GET_NUMBER_SIGNALS", "OCP_IF_CMD_TRACE_GET_SIGNALS_NAMES", "OCP_IF_CMD_TRACE_GET_NUMBER_TRACES", "OCP_IF_CMD_TRACE_GET_TRACES_NAMES", "OCP_IF_CMD_TRACE_GET_ADDRESS", "OCP_IF_CMD_CS_STATUS", "OCP_IF_CMD_CS_ENABLE", "OCP_IF_CMD_CS_DISABLE", "OCP_IF_CMD_CS_CONTROLLER_IF", "OCP_IF_CMD_CS_HARDWARE_IF", "OCP_IF_CMD_CS_GET_NUMBER_CONTROLLERS", "OCP_IF_CMD_CS_GET_CONTROLLERS_NAMES", "OCP_IF_CMD_PLATFORM_ID", "OCP_IF_CMD_PLATFORM_IF", "OCP_IF_CMD_OPIL_UPDATE_MEASUREMENTS", "OCP_IF_CMD_OPIL_UPDATE_SIM_DATA", "OCP_IF_CMD_OPIL_RUN_CONTROL", "OCP_IF_CMD_OPIL_INITIALIZE_CONTROL", "OCP_IF_CMD_OPIL_GET_CONTROL", "OCP_IF_CMD_OPIL_GET_CONTROLLER_DATA", "OCP_IF_CMD_END"] ("CMD")
                    n145 = call "Fc_TCP_Client_33.vi"("CMD"=w385, "Input Cluster"=w380, "error in (no error)"=w386, "Comunication Cluster"=w381) -> ("Output cluster"=w384:T9, "error out"=w382:errorcluster)  [unwired: 4 in, 1 out]
                    n146 = Unbundle By Name(w384) -> ("NB_TRACED_SIGNALS"=w383:i32)
                  }
                  frame #2 {
                    w391 = 5 items=["OCP_IF_CMD_TRACE_READ", "OCP_IF_CMD_TRACE_RESET", "OCP_IF_CMD_TRACE_GET_SIZE", "OCP_IF_CMD_TRACE_SET_SIZE", "OCP_IF_CMD_TRACE_GET_NUMBER_SIGNALS", "OCP_IF_CMD_TRACE_GET_SIGNALS_NAMES", "OCP_IF_CMD_TRACE_GET_NUMBER_TRACES", "OCP_IF_CMD_TRACE_GET_TRACES_NAMES", "OCP_IF_CMD_TRACE_GET_ADDRESS", "OCP_IF_CMD_CS_STATUS", "OCP_IF_CMD_CS_ENABLE", "OCP_IF_CMD_CS_DISABLE", "OCP_IF_CMD_CS_CONTROLLER_IF", "OCP_IF_CMD_CS_HARDWARE_IF", "OCP_IF_CMD_CS_GET_NUMBER_CONTROLLERS", "OCP_IF_CMD_CS_GET_CONTROLLERS_NAMES", "OCP_IF_CMD_PLATFORM_ID", "OCP_IF_CMD_PLATFORM_IF", "OCP_IF_CMD_OPIL_UPDATE_MEASUREMENTS", "OCP_IF_CMD_OPIL_UPDATE_SIM_DATA", "OCP_IF_CMD_OPIL_RUN_CONTROL", "OCP_IF_CMD_OPIL_INITIALIZE_CONTROL", "OCP_IF_CMD_OPIL_GET_CONTROL", "OCP_IF_CMD_OPIL_GET_CONTROLLER_DATA", "OCP_IF_CMD_END"] ("CMD")
                    n147 = call "Fc_TCP_Client_33.vi"("CMD"=w391, "Input Cluster"=w389, "error in (no error)"=w392, "Comunication Cluster"=w390) -> ("Output cluster"=w395:T9, "error out"=w393:errorcluster)  [unwired: 4 in, 1 out]
                    n148 = call <vilib>:"Simple Error Handler.vi"("error in (no error)"=w393) -> ()  [unwired: 4 in, 5 out]
                    n149 = Unbundle By Name(w395) -> ("NAMES TRACED SIGNALS"=w394:string[])
                    n150 = Bundle By Name(cluster=w397, "NB_SIGNALS"=w388, "SIGNALS_NAMES"=w394) -> (w396:T3)
                    n151 = shared-variable ".\\Share_Variables.lvlib\\Signals_name"(w394) -> ()  [unwired: 1 in, 1 out]
                    n152 = shared-variable ".\\Share_Variables.lvlib\\number_signals"(w388) -> ()  [unwired: 1 in, 1 out]
                  }
                }
              }
            }
            n153 = shared-variable ".\\Share_Variables.lvlib\\Mode_signal_conf"("Mode") -> ()  [unwired: 1 in, 1 out]
            n154 = case shown="\"Item 1\"" "Mode" {
              tunnel: [200 ("Refresh time (sec)") w399] -> w346
              frame "Item 1" {
              }
              frame "Item 0", Default {
                n155 = Multiply(x=1, y="Refresh time (ms)") -> (x*y=w399:i32)
              }
            }
            n156 = Bundle By Name(cluster=w341, "Refresh time ms"=w346, "Mode"="Mode", "Start"=TRUE) -> (w348:T3)
          }
        }
      }
      event "Trace names": Value Change {
        n157 = event-data() -> ()  [unwired: 1 in, 6 out]
        n158 = property on="Trace names" class="CmbBox"() -> ("Value"=w406:string, "Strings[]"=w405:string[])  [unwired: 2 in, 2 out]
        n159 = Search 1D Array(1D array=w405, element=w406) -> (index of element=w404:i32)  [unwired: 1 in]
        n160 = Unbundle By Name(w414) -> ("Port"=w412:i32, "hostname"=w411:string, "timeout ms"=w410:i32)
        n161 = To Long Integer(number=w404) -> (32bit integer=w403:i32)
        n162 = call "TCP Client_32.vi"("CMD"=2, "remote port \nor service name"=w412, "ID_Trace"=w403, "timeout ms"=w410, "Address"=w411) -> ("Output cluster"=w409:T10, "error out"=w407:errorcluster)  [unwired: 3 in, 1 out]
        n163 = call <vilib>:"Simple Error Handler.vi"("error in (no error)"=w407) -> ()  [unwired: 4 in, 5 out]
        n164 = Unbundle By Name(w409) -> ("TRACE_SIZE"=w408:i32)
        n165 = property on="Size bytes" class="DigNum (strict)"("Value"=w408) -> ()  [unwired: 2 in, 2 out]
      }
      event "# Control": Value Change {
        n166 = event-data() -> ()  [unwired: 1 in, 6 out]
        n167 = Unbundle By Name(w422) -> ("Port"=w416:i32, "hostname"=w418:string, "timeout ms"=w417:i32)
        n168 = Bundle By Name(cluster=w421, "timeout ms"=w417, "remote port"=w416, "Address"=w418) -> (w419:T6)
        n169 = flat-sequence {
          tunnel: w420 -> [w428]
          tunnel: w419 -> [w425]
          tunnel: [w423] -> w415
          frame #0 {
            w427 = 9 items=["OCP_IF_CMD_TRACE_READ", "OCP_IF_CMD_TRACE_RESET", "OCP_IF_CMD_TRACE_GET_SIZE", "OCP_IF_CMD_TRACE_SET_SIZE", "OCP_IF_CMD_TRACE_GET_NUMBER_SIGNALS", "OCP_IF_CMD_TRACE_GET_SIGNALS_NAMES", "OCP_IF_CMD_TRACE_GET_NUMBER_TRACES", "OCP_IF_CMD_TRACE_GET_TRACES_NAMES", "OCP_IF_CMD_TRACE_GET_ADDRESS", "OCP_IF_CMD_CS_STATUS", "OCP_IF_CMD_CS_ENABLE", "OCP_IF_CMD_CS_DISABLE", "OCP_IF_CMD_CS_CONTROLLER_IF", "OCP_IF_CMD_CS_HARDWARE_IF", "OCP_IF_CMD_CS_GET_NUMBER_CONTROLLERS", "OCP_IF_CMD_CS_GET_CONTROLLERS_NAMES", "OCP_IF_CMD_PLATFORM_ID", "OCP_IF_CMD_PLATFORM_IF", "OCP_IF_CMD_OPIL_UPDATE_MEASUREMENTS", "OCP_IF_CMD_OPIL_UPDATE_SIM_DATA", "OCP_IF_CMD_OPIL_RUN_CONTROL", "OCP_IF_CMD_OPIL_INITIALIZE_CONTROL", "OCP_IF_CMD_OPIL_GET_CONTROL", "OCP_IF_CMD_OPIL_GET_CONTROLLER_DATA", "OCP_IF_CMD_END"] ("CMD")
            n170 = property on="# Control" class="CmbBox"() -> ("Value"=w431:string, "Strings[]"=w432:string[])  [unwired: 2 in, 2 out]
            n171 = Search 1D Array(1D array=w432, element=w431) -> (index of element=w430:i32)  [unwired: 1 in]
            n172 = To Long Integer(number=w430) -> (32bit integer=w429:i32)
            n173 = Bundle By Name(cluster=w428, "CS_ID"=w429) -> (w424:T5)
            n174 = call "Fc_TCP_Client_33.vi"("CMD"=w427, "Input Cluster"=w424, "Comunication Cluster"=w425) -> ("Output cluster"=w433:T9, "error out"=w423:errorcluster)  [unwired: 5 in, 1 out]
            n175 = Unbundle By Name(w433) -> ("CS STATUS"=→"Current CS status":i32)
          }
        }
        n176 = call <vilib>:"Simple Error Handler.vi"("error in (no error)"=w415) -> ()  [unwired: 4 in, 5 out]
      }
      event "CS enable": Value Change {
        n177 = event-data() -> ()  [unwired: 1 in, 6 out]
        n178 = Unbundle By Name(w446) -> ("Port"=w440:i32, "hostname"=w442:string, "timeout ms"=w441:i32)
        n179 = Bundle By Name(cluster=w445, "timeout ms"=w441, "remote port"=w440, "Address"=w442) -> (w443:T6)
        n180 = flat-sequence {
          tunnel: w444 -> [w452]
          tunnel: w443 -> [w450]
          tunnel: ["CS enable"] -> w439
          tunnel: [w450] -> w438
          tunnel: [w449] -> w437
          tunnel: [T5 {"TRACE_SIZE"=0, "CS_ID"=0, "TRACE ID"=0, "CMD"=0, "DATA(M)"=0} ("Input Cluster")] -> w435
          tunnel: [w447] -> w434
          tunnel: w439 -> [w462]
          tunnel: w438 -> [w461]
          tunnel: w437 -> [w460]
          tunnel: [w458] -> w436
          tunnel: w435 -> [w457]
          tunnel: w434 -> [w456]
          frame #0 {
            n181 = property on="# Control" class="CmbBox"() -> ("Value"=w454:string, "Strings[]"=w455:string[])  [unwired: 2 in, 2 out]
            n182 = Search 1D Array(1D array=w455, element=w454) -> (index of element=w453:i32)  [unwired: 1 in]
            n183 = To Long Integer(number=w453) -> (32bit integer=w447:i32)
            n184 = Bundle By Name(cluster=w452, "CS_ID"=w447) -> (w449:T5)
          }
          frame #1 {
            n185 = case shown="True" w462 {
              selector: w462 -> [w467 w475]
              tunnel: w461 -> [w465 w474]
              tunnel: w460 -> [w466 _]
              tunnel: [w467 w475] -> w459
              tunnel: [w463 w473] -> w458
              tunnel: w457 -> [_ w472]
              tunnel: w456 -> [_ w470]
              frame False {
                w464 = 11 items=["OCP_IF_CMD_TRACE_READ", "OCP_IF_CMD_TRACE_RESET", "OCP_IF_CMD_TRACE_GET_SIZE", "OCP_IF_CMD_TRACE_SET_SIZE", "OCP_IF_CMD_TRACE_GET_NUMBER_SIGNALS", "OCP_IF_CMD_TRACE_GET_SIGNALS_NAMES", "OCP_IF_CMD_TRACE_GET_NUMBER_TRACES", "OCP_IF_CMD_TRACE_GET_TRACES_NAMES", "OCP_IF_CMD_TRACE_GET_ADDRESS", "OCP_IF_CMD_CS_STATUS", "OCP_IF_CMD_CS_ENABLE", "OCP_IF_CMD_CS_DISABLE", "OCP_IF_CMD_CS_CONTROLLER_IF", "OCP_IF_CMD_CS_HARDWARE_IF", "OCP_IF_CMD_CS_GET_NUMBER_CONTROLLERS", "OCP_IF_CMD_CS_GET_CONTROLLERS_NAMES", "OCP_IF_CMD_PLATFORM_ID", "OCP_IF_CMD_PLATFORM_IF", "OCP_IF_CMD_OPIL_UPDATE_MEASUREMENTS", "OCP_IF_CMD_OPIL_UPDATE_SIM_DATA", "OCP_IF_CMD_OPIL_RUN_CONTROL", "OCP_IF_CMD_OPIL_INITIALIZE_CONTROL", "OCP_IF_CMD_OPIL_GET_CONTROL", "OCP_IF_CMD_OPIL_GET_CONTROLLER_DATA", "OCP_IF_CMD_END"] ("CMD")
                n186 = call "Fc_TCP_Client_33.vi"("CMD"=w464, "Input Cluster"=w466, "Comunication Cluster"=w465) -> ("error out"=w463:errorcluster)  [unwired: 5 in, 2 out]
              }
              frame True {
                w469 = 10 items=["OCP_IF_CMD_TRACE_READ", "OCP_IF_CMD_TRACE_RESET", "OCP_IF_CMD_TRACE_GET_SIZE", "OCP_IF_CMD_TRACE_SET_SIZE", "OCP_IF_CMD_TRACE_GET_NUMBER_SIGNALS", "OCP_IF_CMD_TRACE_GET_SIGNALS_NAMES", "OCP_IF_CMD_TRACE_GET_NUMBER_TRACES", "OCP_IF_CMD_TRACE_GET_TRACES_NAMES", "OCP_IF_CMD_TRACE_GET_ADDRESS", "OCP_IF_CMD_CS_STATUS", "OCP_IF_CMD_CS_ENABLE", "OCP_IF_CMD_CS_DISABLE", "OCP_IF_CMD_CS_CONTROLLER_IF", "OCP_IF_CMD_CS_HARDWARE_IF", "OCP_IF_CMD_CS_GET_NUMBER_CONTROLLERS", "OCP_IF_CMD_CS_GET_CONTROLLERS_NAMES", "OCP_IF_CMD_PLATFORM_ID", "OCP_IF_CMD_PLATFORM_IF", "OCP_IF_CMD_OPIL_UPDATE_MEASUREMENTS", "OCP_IF_CMD_OPIL_UPDATE_SIM_DATA", "OCP_IF_CMD_OPIL_RUN_CONTROL", "OCP_IF_CMD_OPIL_INITIALIZE_CONTROL", "OCP_IF_CMD_OPIL_GET_CONTROL", "OCP_IF_CMD_OPIL_GET_CONTROLLER_DATA", "OCP_IF_CMD_END"] ("CMD")
                n187 = Bundle By Name(cluster=w472, "CS_ID"=w470) -> (w471:T5)
                n188 = call "TCP Client_34_enablep.vi"("CMD"=w469, "CS_IF_Params"="CS_IF_Cluster 2", "Input Cluster"=w471, "Comunication Cluster"=w474) -> ("error out"=w473:errorcluster)  [unwired: 4 in, 2 out]
              }
            }
            "Enable?" <- w459
          }
        }
        n189 = call <vilib>:"Simple Error Handler.vi"("error in (no error)"=w436) -> ()  [unwired: 4 in, 5 out]
      }
    }
    n190 = Dequeue Element(queue=w54, timeout in ms (-1)=100, error in (no error)=w50) -> (queue out=w51:refnum<queue>, element=w53:string, timed out?=w52:bool, error out=w44:errorcluster)
    n191 = property on="Multicolumn Listbox" class="MCListbox (strict)"() -> ("ItemNames"=w42:string[][])  [unwired: 2 in, 2 out]
    n192 = case shown="False" w52 {
      tunnel: w53 -> [w85 _]
      frame False {
        n193 = Match Pattern(string=w85, regular expression="::") -> (before substring=w84:string, after substring=w83:string)  [unwired: 1 in, 2 out]
        n194 = case shown="\"process started\"" w84 {
          tunnel: w83 -> [_ w95 w100]
          frame "False", Default {
            # "unhandled received commands."
            n195 = call <vilib>:"Error Cluster From Error Code.vi"("error message (\"\")"="Invalid command received from process VI" ("error message (\"\")"), "error code (0)"=1) -> ("error out"=w87:errorcluster)  [unwired: 7 in]
            n196 = call <vilib>:"Simple Error Handler.vi"("error in (no error)"=w87) -> ()  [unwired: 4 in, 5 out]
          }
          frame "process stopped" {
            n197 = property on="Multicolumn Listbox" class="MCListbox (strict)"() -> ("ItemNames"=w91:string[][])  [unwired: 2 in, 2 out]
            n198 = Index Array(array=w91, index (col)=0 ("disabled index (col)")) -> (element=w92:string[])  [unwired: 1 in]
            n199 = Search 1D Array(1D array=w92, element=w95) -> (index of element=w93:i32)  [unwired: 1 in]
            n200 = Delete From Array(array=w91, index (row)=w93) -> (array with subset deleted=w90:string[][])  [unwired: 2 in, 1 out]
            n201 = property on="Multicolumn Listbox" class="MCListbox (strict)"("ItemNames"=w90) -> ()  [unwired: 2 in, 2 out]
          }
          frame "process started" {
            n202 = Build Array(w100, "" ("element")) -> (w98:string[])
            n203 = property on="Multicolumn Listbox" class="MCListbox (strict)"() -> ("ItemNames"=w97:string[][])  [unwired: 2 in, 2 out]
            n204 = Build Array (concatenate)(w97, w98) -> (w96:string[][])
            n205 = property on="Multicolumn Listbox" class="MCListbox (strict)"("ItemNames"=w96) -> ()  [unwired: 2 in, 2 out]
          }
        }
      }
      frame True {
      }
    }
    n206 = Index Array(array=w39, index=0) -> (element=w38:refnum<queue>)
    n207 = case shown="False" "Send message" {
      tunnel: w42 -> [_ w60]
      tunnel: w41 -> [_ w62]
      tunnel: w38 -> [_ w61]
      frame False {
      }
      frame True {
        n208 = Array Size(array=w60) -> (size(s)=w58:i32[])
        n209 = Index Array(array=w58, index=0) -> (element=w57:i32)
        n210 = property on="Process 2" class="DigNum (strict)"("Maximum"=w57) -> ()  [unwired: 2 in, 2 out]
        n211 = case shown="Default" "Process 2" {
          selector: "Process 2" -> [w80 _]
          tunnel: w60 -> [w82 _]
          tunnel: w62 -> [w70 _]
          tunnel: w61 -> [w71 _]
          frame Default {
            w66 = FALSE ("create if not found? (T)")
            n212 = Index Array(array=w82, index (row)=w80, index (col)=0 ("disabled index (col)")) -> (element=w64:string)
            n213 = Get Queue Status(queue=w71, error in (no error)=w70) -> (error out=w68:errorcluster)  [unwired: 1 in, 7 out]
            n214 = local write "Send message"(w66) -> ()
            n215 = Obtain Queue(name (unnamed)=w64, element data type="", create if not found? (T)=w66, error in (no error)=w68) -> (queue out=w69:refnum<queue>, error out=w67:errorcluster)  [unwired: 1 in, 1 out]
            n216 = Concatenate Strings("message::", "msj") -> (w75:string)
            n217 = Get Queue Status(queue=w69, error in (no error)=w67) -> (queue out=w79:refnum<queue>, error out=w78:errorcluster)  [unwired: 1 in, 6 out]
            n218 = Enqueue Element(queue=w79, element=w75, error in (no error)=w78) -> (queue out=w74:refnum<queue>, error out=w73:errorcluster)  [unwired: 1 in, 1 out]
            n219 = Release Queue(queue=w74, error in (no error)=w73) -> (error out=w72:errorcluster)  [unwired: 1 in, 2 out]
            n220 = call <vilib>:"Simple Error Handler.vi"("error in (no error)"=w72) -> ()  [unwired: 4 in, 5 out]
          }
          frame ..-1 {
          }
        }
      }
    }
  }
  n221 = Flush Queue(queue=w18) -> ()  [unwired: 1 in, 3 out]
  n222 = for {
    tunnel: w32 -> [w477] mode=indexing
    n223 = Release Queue(queue=w477, force destroy? (F)=FALSE) -> ()  [unwired: 1 in, 3 out]
  }
  n224 = Release Queue(queue=w18, error in (no error)=w27) -> (error out=w25:errorcluster)  [unwired: 1 in, 2 out]
  n225 = property on="Multicolumn Listbox" class="MCListbox (strict)"(error in=w25) -> (error out=w21:errorcluster, "ItemNames"=w24:string[][])  [unwired: 1 in, 1 out]
  n226 = Index Array(array=w24, index (col)=0 ("disabled index (col)")) -> (element=w22:string[])  [unwired: 1 in]
  n227 = for {
    tunnel: w22 -> [w487] mode=indexing
    shift-right: [w484] -> w20
    shift-left: w21 -> [w486]
    n228 = Obtain Queue(name (unnamed)=w487, element data type="", error in (no error)=w486) -> (queue out=w479:refnum<queue>, error out=w481:errorcluster)  [unwired: 2 in, 1 out]
    n229 = Enqueue Element(queue=w479, element="exit::", error in (no error)=w481) -> (queue out=w478:refnum<queue>, error out=w480:errorcluster)  [unwired: 1 in, 1 out]
    n230 = Release Queue(queue=w478, force destroy? (F)=FALSE, error in (no error)=w480) -> (error out=w484:errorcluster)  [unwired: 2 out]
  }
  n231 = call <vilib>:"Simple Error Handler.vi"("error in (no error)"=w20) -> ("error out"=w19:errorcluster)  [unwired: 4 in, 4 out]
  n232 = flat-sequence {
    tunnel: w19 -> [_]
    frame #0 {
      n233 = property class="App"() -> ("App.Kind"=w490:T11)  [unwired: 2 in, 2 out]
      n234 = Equal?(x=w490, y=T11."Run Time System" ("Application:Kind")) -> (x = y?=→"Close":bool)
    }
  }
